vi "set(byVal).vi"(10 "UniqueName in":refnum<class "UniqueName.lvclass">, 11 "NameRegistry in":refnum<class "NameRegistry.lvclass">) -> (1 "Replaced?":bool, 2 "UniqueName out":refnum<class "UniqueName.lvclass">, 3 "NameRegistry out":refnum<class "NameRegistry.lvclass">)   [LabVIEW 2013, in "UniqueName.lvlib" / "NameRegistry.lvclass"]
uses:
  NameRegistry.lvclass
  UniqueNameClass/UniqueName.lvclass
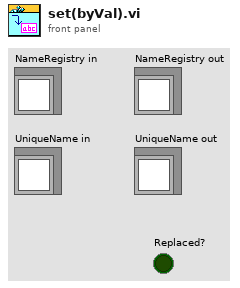
[diagram p1: front panel]
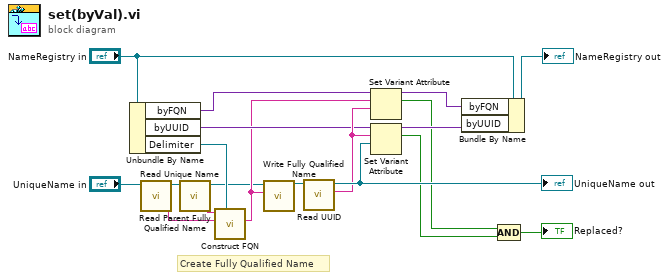
[diagram p0: block diagram]
diagram:
  # "Create Fully Qualified Name"
  n1 = Unbundle By Name("NameRegistry in") -> ("byFQN"=w12:variant, "byUUID"=w15:variant, "Delimiter"=w10:refnum<class "Delimiter.lvclass">)
  n2 = call "Read Unique Name.vi"("UniqueName in"="UniqueName in") -> ("Unique Name"=w8:string, "UniqueName out"=w7:refnum<class "UniqueName.lvclass">)  [unwired: 9 in]
  n3 = call "Read Parent Fully Qualified Name.vi"("UniqueName in"=w7) -> ("Parent Fully Qualified Name"=w5:string, "UniqueName out"=w6:refnum<class "UniqueName.lvclass">)  [unwired: 9 in]
  n4 = call "Construct FQN.vi"("Delimiter"=w10, "Name"=w8, "Parent FQN"=w5) -> ("FQN"=w13:string)  [unwired: 8 in]
  n5 = call "Write Fully Qualified Name.vi"("Fully Qualified Name"=w13, "UniqueName in"=w6) -> ("UniqueName out"=w14:refnum<class "UniqueName.lvclass">)  [unwired: 9 in]
  n6 = call "Read UUID.vi"("UniqueName in"=w14) -> ("UUID"=w18:string, "UniqueName out"=w19:refnum<class "UniqueName.lvclass">)  [unwired: 9 in]
  "UniqueName out" <- w19
  n7 = Set Variant Attribute(Variant=w12, name=w13, value=w18) -> (Variant out=w17:variant, replaced=w2:bool)  [unwired: 1 in, 1 out]
  n8 = Set Variant Attribute(Variant=w15, name=w18, value=w19) -> (Variant out=w16:variant, replaced=w3:bool)  [unwired: 1 in, 1 out]
  n9 = Bundle By Name(cluster="NameRegistry in", "byFQN"=w17, "byUUID"=w16) -> (→"NameRegistry out":refnum<class "NameRegistry.lvclass">)
  n10 = Compound Arithmetic op=AND(w2, w3) -> (→"Replaced?":bool)
